vi "ApplyLayoutToObject.vi"(5 "scaling settings":T1={"scaling factor"={"horizontal"=1.0, "vertical"=1.0}, "scale text"=FALSE} {"scaling factor"."vertical" min=0.0; "scaling factor"."horizontal" min=0.0}, 7 "properties to ignore":variant, 8 "error in (no error)":errorcluster, 10 "GObj Refnum":refnum<vi>, 11 "String Control Layout in":refnum<class "String Control Layout.lvclass">) -> (0 "error out":errorcluster, 3 "String Control Layout out":refnum<class "String Control Layout.lvclass">)   [LabVIEW 2010, in "NI_SE_Front Panel Layout.lvlib" / "String Control Layout.lvclass"]
doc: "Apply layout information to the GObj Refnum."
uses:
  String Control Layout.lvclass
  NI_SE_Front Panel Layout.lvlib
  Object Layout/Object Layout.lvclass
  Control Layout/Control Layout.lvclass
  XY Scaling Factor.ctl
  Scaling Factor_Options.ctl
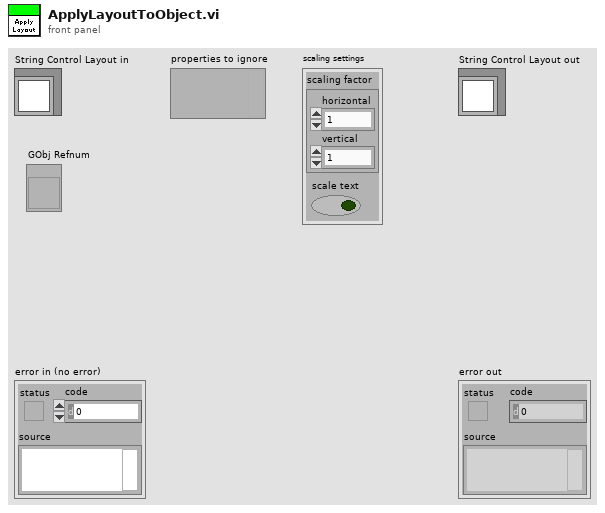
[diagram p1: front panel]
types:
  T1 = typedef "NI_SE_Front Panel Layout.lvlib/Scaling Factor_Options.ctl" = cluster{"scaling factor":T2, "scale text":bool}
  T2 = typedef "NI_SE_Front Panel Layout.lvlib/XY Scaling Factor.ctl" = cluster{"horizontal":dbl, "vertical":dbl}
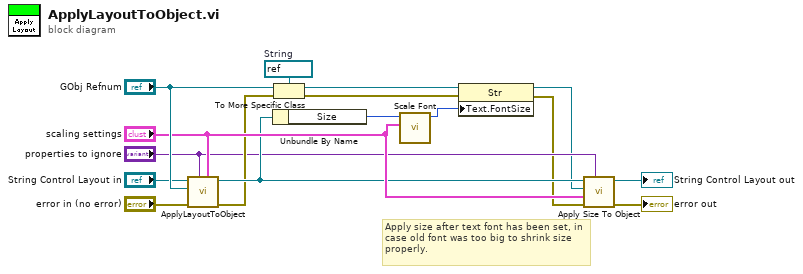
[diagram p0: block diagram]
diagram:
  w7 = refnum<vi> refnum  # String
  # "Apply size after text font has been set, in case old font was too big to shrink size properly."
  n1 = call-parent "ApplyLayoutToObject.vi"("scaling settings"="scaling settings", "properties to ignore"="properties to ignore", "error in (no error)"="error in (no error)", "GObj Refnum"="GObj Refnum", "Control Layout in"="String Control Layout in") -> ("error out"=w11:errorcluster, "Control Layout out"=w12:refnum<class "String Control Layout.lvclass">)  [unwired: 5 in]
  n2 = Unbundle By Name(w12) -> ("Size"=w4:u16)
  n3 = To More Specific Class(target class=w7, reference="GObj Refnum", error in=w11) -> (specific class reference=w6:refnum<vi>, error out=w5:errorcluster)
  n4 = call "Scale Font.vi"("scaling settings"="scaling settings", "font size in"=w4) -> ("font size out"=w3:u16)  [unwired: 9 in]
  n5 = property class="Str"(reference=w6, error in=w5, "Text.FontSize"=w3) -> (reference out=w1:refnum<vi>, error out=w2:errorcluster)
  n6 = call "Apply Size To Object.vi"("properties to ignore"="properties to ignore", "error in (no error)"=w2, "scaling settings"="scaling settings", "GObj Refnum"=w1, "NI_SE_Object Layout in"=w12) -> ("error out"=→"error out":errorcluster, "NI_SE_Object Layout out"=→"String Control Layout out":refnum<class "String Control Layout.lvclass">)  [unwired: 5 in]
